vi "Edit Instrument Tag With New Config.vi"(6 "Tree":string, 7 "Name":string(combo), 8 "error in (no error)":errorcluster, 9 "Channel #":u16, 10 "Visa Resource":refnum<visa-resource-name> caption="VISA Resource", 11 "TreeControl in":refnum<vi>) -> (0 "error out":errorcluster, 1 "New Configuration?":bool, 3 "TreeControl out":refnum<vi>)   [LabVIEW 2018]
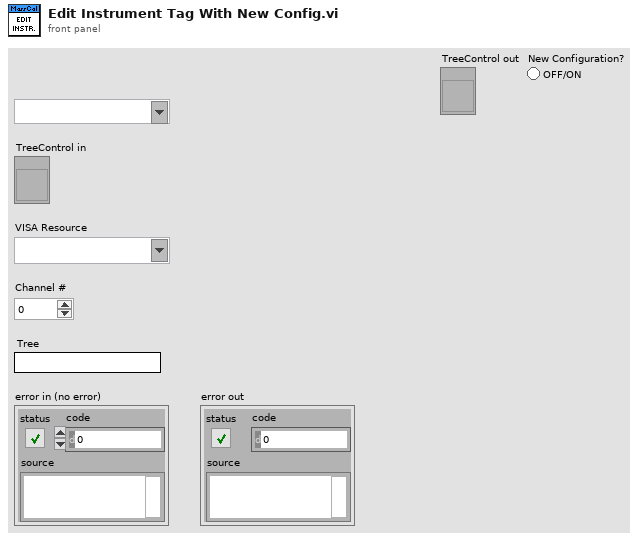
[diagram p1: front panel]
types:
  T1 = typedef "Test Manager Tree Tag.ctl" = cluster{"ItemType":T2, "VISA Resource":refnum<visa-resource-name>, "Name":string, "Channel #":u16, "ComparatorID":u16, "UIMod_ID":i16}
  T2 = typedef "Tree Item Type.ctl" = enum16{"Comparator", "Temp Group", "Press Group", "Hygro Group", "Thermometer", "PressureTransducer", "Hygrometers", "Add Comparator", "Add Thermometer", "Add Barometer", "Add Hygrometer"}
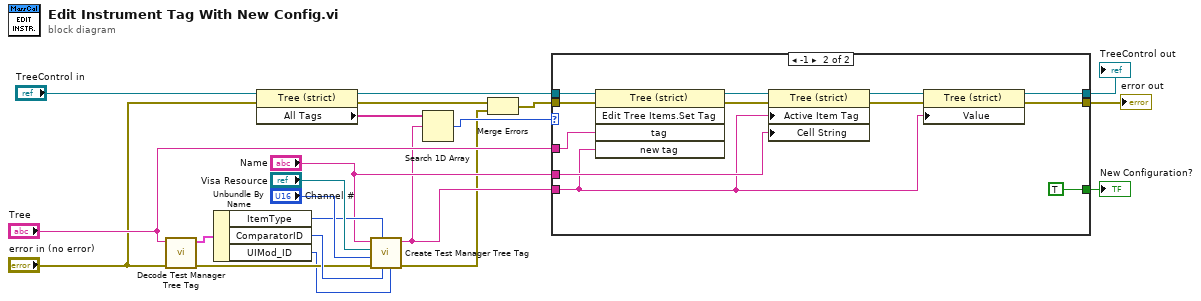
[diagram p0: block diagram]
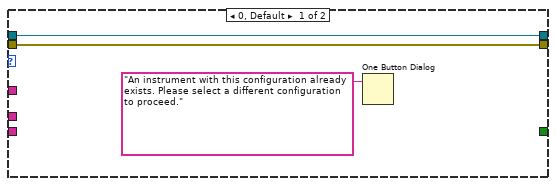
[diagram p2: hidden frame]
diagram:
  n1 = call "Decode Test Manager Tree Tag.vi"("error in (no error)"="error in (no error)", "Tag"="Tree") -> ("error out"=w14:errorcluster, "Test Manager Tree Tag"=w15:T1)  [unwired: 8 in]
  n2 = Unbundle By Name(w15) -> ("ItemType"=w16:T2, "ComparatorID"=w19:u16, "UIMod_ID"=w1:i16)
  n3 = property class="Tree (strict)"(reference="TreeControl in", error in="error in (no error)") -> (reference out=w11:refnum<vi>, error out=w6:errorcluster, "All Tags"=w9:string[])
  n4 = call "Create Test Manager Tree Tag.vi"("UIMod_ID"=w1, "Comparator ID"=w19, "ItemType"=w16, "error in (no error)"=w14, "Channel #"="Channel #", "VISA Resource"="Visa Resource", "Name"="Name") -> ("error out"=w5:errorcluster, "Tag"=w8:string)  [unwired: 2 in, 1 out]
  n5 = Search 1D Array(1D array=w9, element=w8) -> (index of element=w7:i32)  [unwired: 1 in]
  n6 = Merge Errors(w6, w5) -> (w4:errorcluster)
  n7 = case shown="-1" w7 {
    tunnel: "Tree" -> [_ w36]
    tunnel: w4 -> [w24 w35]
    tunnel: [w24 w29] -> w13
    tunnel: "Name" -> [_ w31]
    tunnel: w11 -> [w22 w30]
    tunnel: w8 -> [_ w27]
    tunnel: [w22 w26] -> w3
    tunnel: [_ TRUE] -> w2
    frame 0, Default {
      n8 = One Button Dialog(message="An instrument with this configuration already exists. Please select a different configuration to proceed.") -> ()  [unwired: 1 in, 1 out]
    }
    frame -1 {
      n9 = invoke class="Tree (strict)" method="Edit Tree Items.Set Tag"(reference=w30, error in=w35, "tag"=w36, "new tag"=w27) -> (reference out=w32:refnum<vi>, error out=w34:errorcluster)  [unwired: 1 in, 3 out]
      n10 = property class="Tree (strict)"(reference=w32, error in=w34, "Active Item Tag"=w27, "Cell String"=w31) -> (reference out=w28:refnum<vi>, error out=w33:errorcluster)
      n11 = property class="Tree (strict)"(reference=w28, error in=w33, "Value"=w27) -> (reference out=w26:refnum<vi>, error out=w29:errorcluster)
    }
  }
  "error out" <- w13
  "TreeControl out" <- w3
  "New Configuration?" <- w2
